vi "FormProductsCluster.vi"() -> ()   [LabVIEW 2013]
panel:
  in  "功能选择":T1
  in  "选项卡控件":T2(tab)
  in  "平均值差":cluster{"limitH":dbl, "unit":string}
  in  "波动值":cluster{"limitH":dbl, "unit":string}
  in  "磨合负载":cluster{"vaule":dbl, "unit":string}
  in  "磨合次数":cluster{"vaule":dbl, "unit":string}
  in  "磨合圈数":cluster{"vaule":dbl, "unit":string}
  in  "检测速度":cluster{"vaule":dbl, "unit":string}
  in  "磨合速度":cluster{"vaule":dbl, "unit":string}
  in  "平均值":T3
  in  "平均值 2":T3
  in  "磨合速度 2":cluster{"vaule":dbl, "unit":string}
  in  "检测速度 2":cluster{"vaule":dbl, "unit":string}
  in  "磨合圈数 2":cluster{"vaule":dbl, "unit":string}
  in  "磨合次数 2":cluster{"vaule":dbl, "unit":string}
  in  "磨合负载 2":cluster{"vaule":dbl, "unit":string}
  in  "波动值 2":cluster{"limitH":dbl, "unit":string}
  in  "平均值差 2":cluster{"limitH":dbl, "unit":string}
  in  "产品选择":bool
  in  "产品删除":bool
  in  "产品更新":bool
  in  "产品注册":bool
  in  "产品":string(combo)
  # "磨合速度"
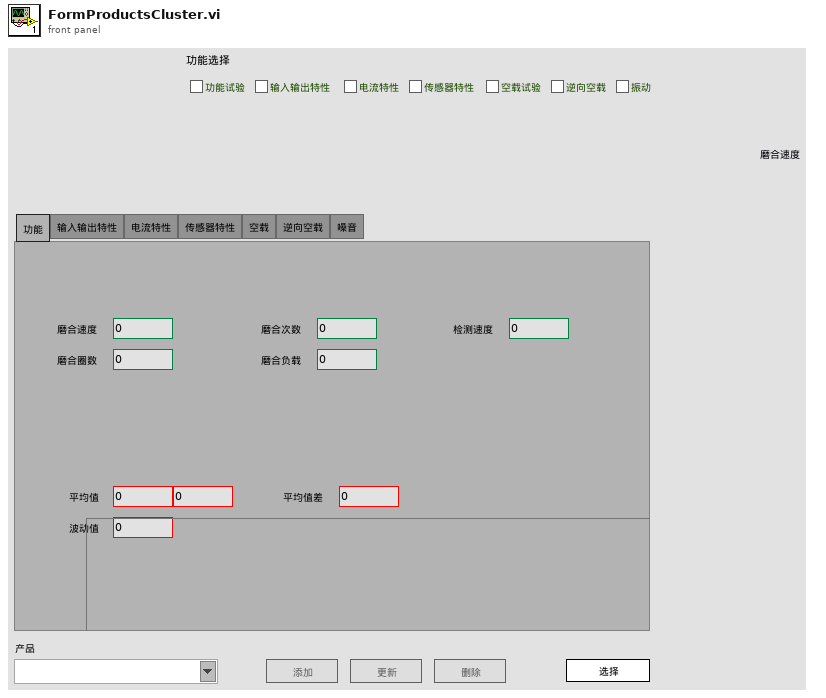
[diagram p1: front panel]
types:
  T1 = cluster{"功能试验":bool, "输入输出特性":bool, "电流特性":bool, "传感器特性":bool, "空载试验":bool, "逆向空载":bool, "振动":bool}
  T2 = enum32{"功能", "输入输出特性", "电流特性", "传感器特性", "空载", "逆向空载", "噪音"}
  T3 = cluster{"limitH":dbl, "limitL":dbl, "unit":string}
  T4 = enum8{"Enabled", "Disabled", "Disabled and Grayed Out"}
  T5 = enum16{"selectdata", "selectsave", "selectlist", "selectshow"}
  T6 = cluster{"userCode":string, "userName":string, "userStatus":string, "connectionMode":string, "takesTime":string, "countDone":string, "countOK":string, "countNG":string, "rigStatus":string, "productsName":string, "partCode1":string, "partCode2":string, "partCode3":string}
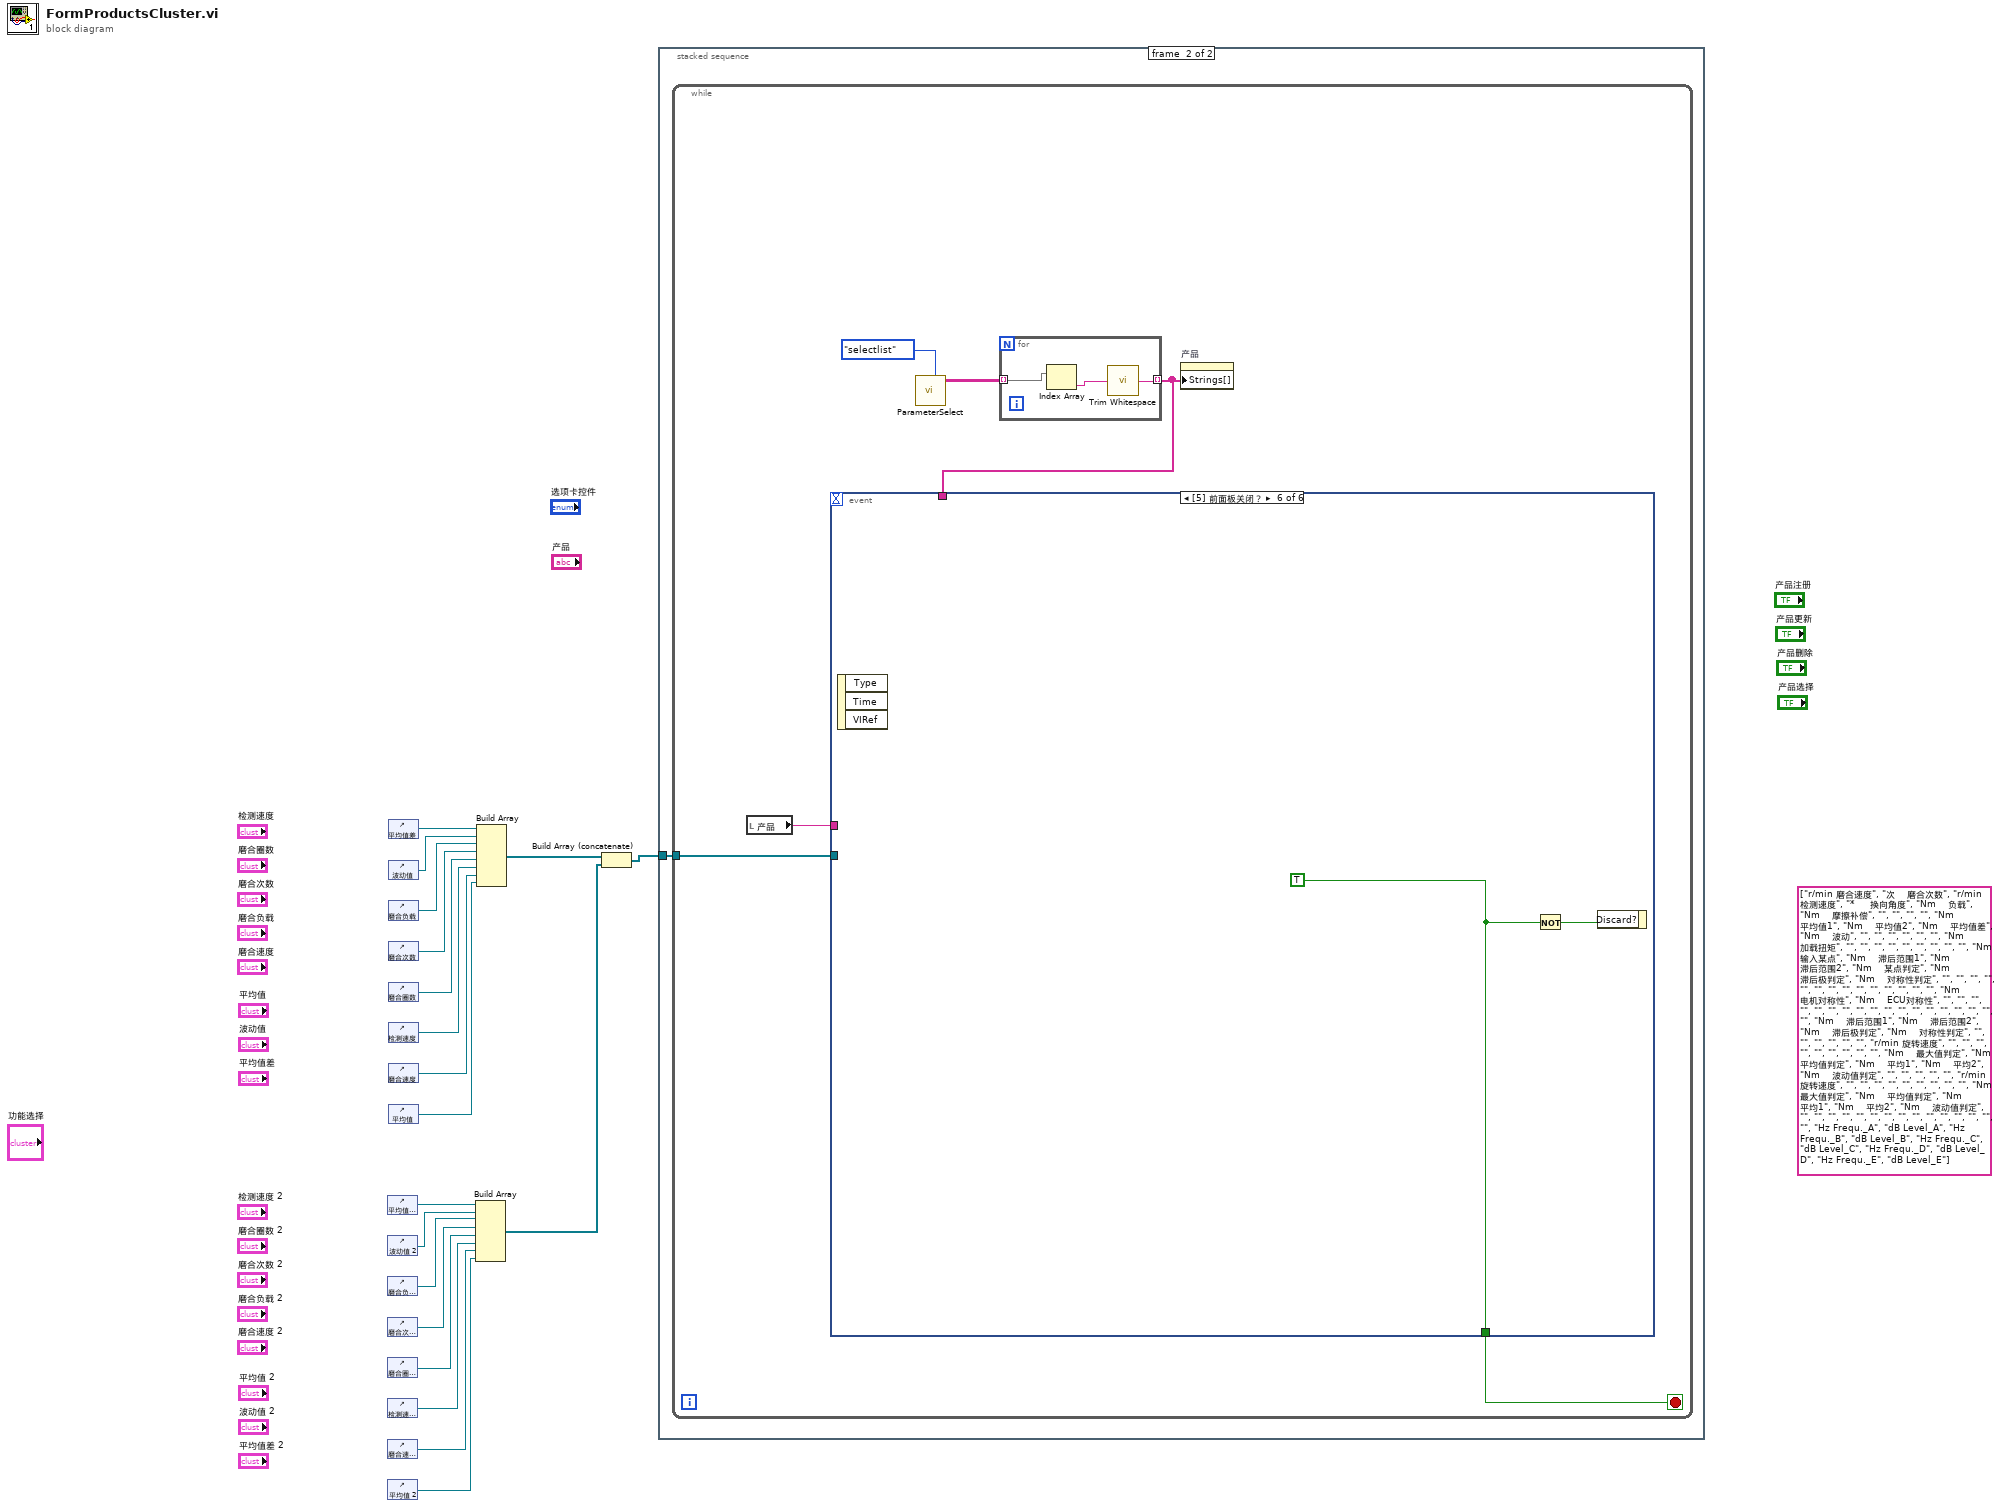
[diagram p0: block diagram]
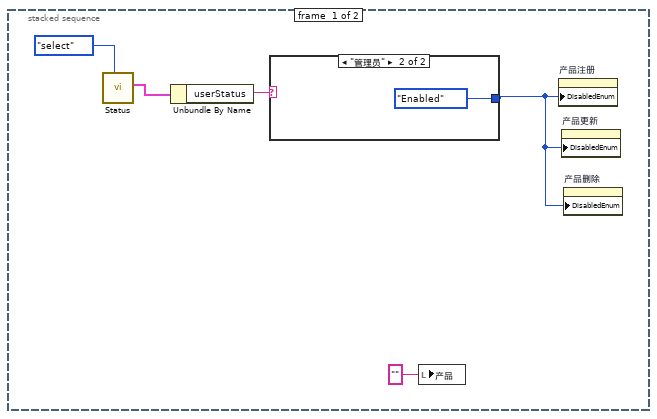
[diagram p2: hidden frame]
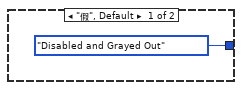
[diagram p3: hidden frame]
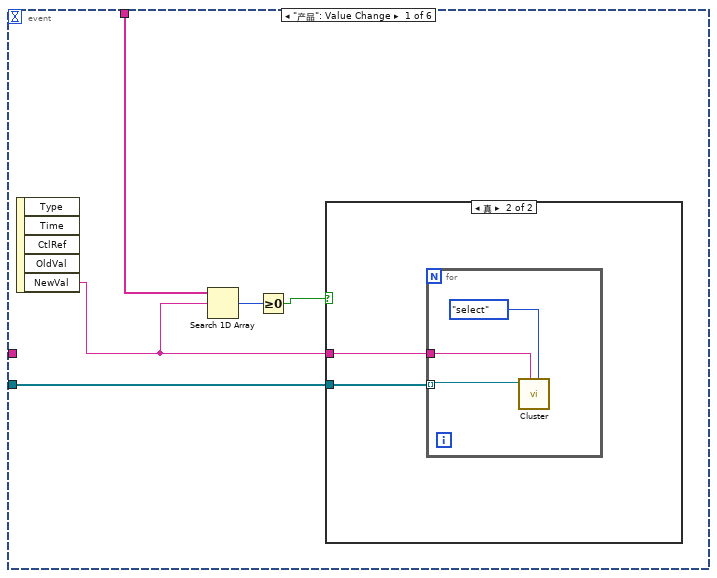
[diagram p4: hidden frame]
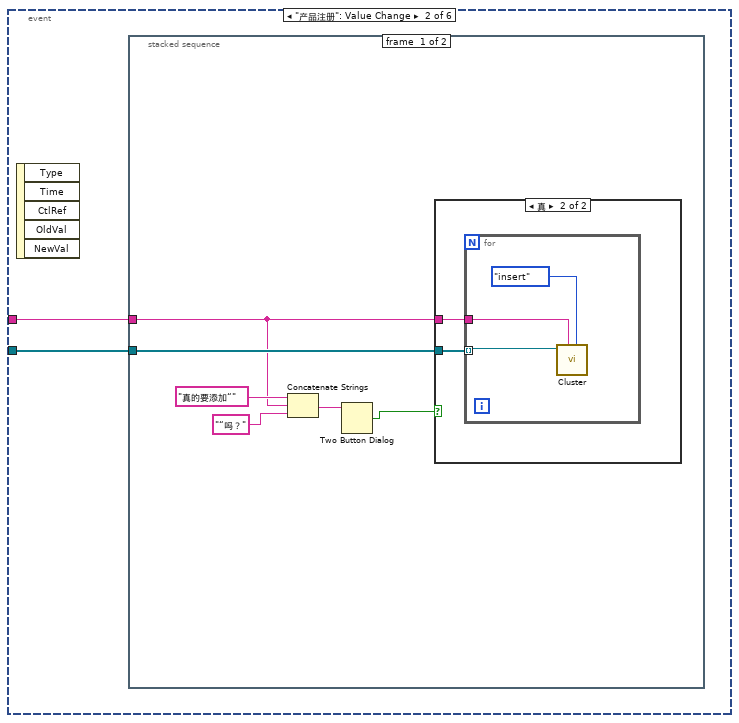
[diagram p6: hidden frame]
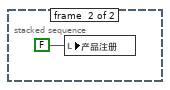
[diagram p8: hidden frame]
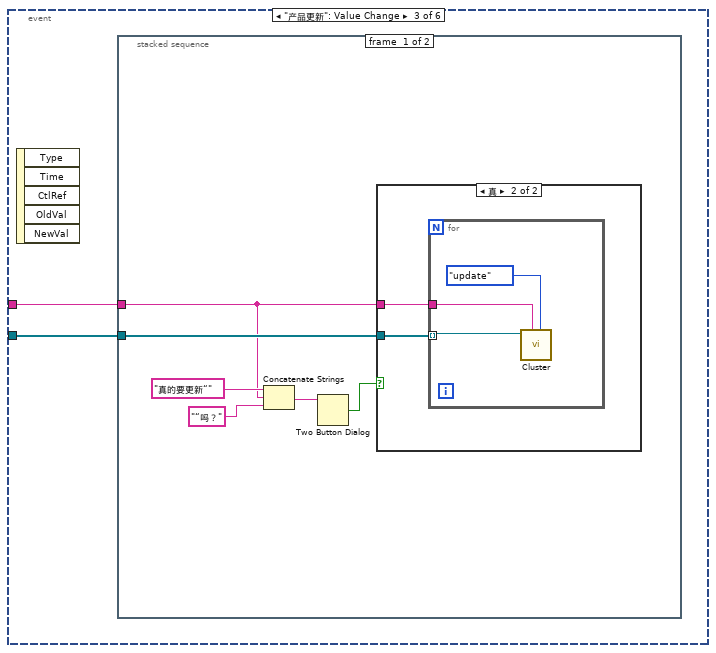
[diagram p9: hidden frame]
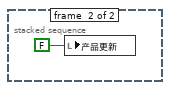
[diagram p11: hidden frame]
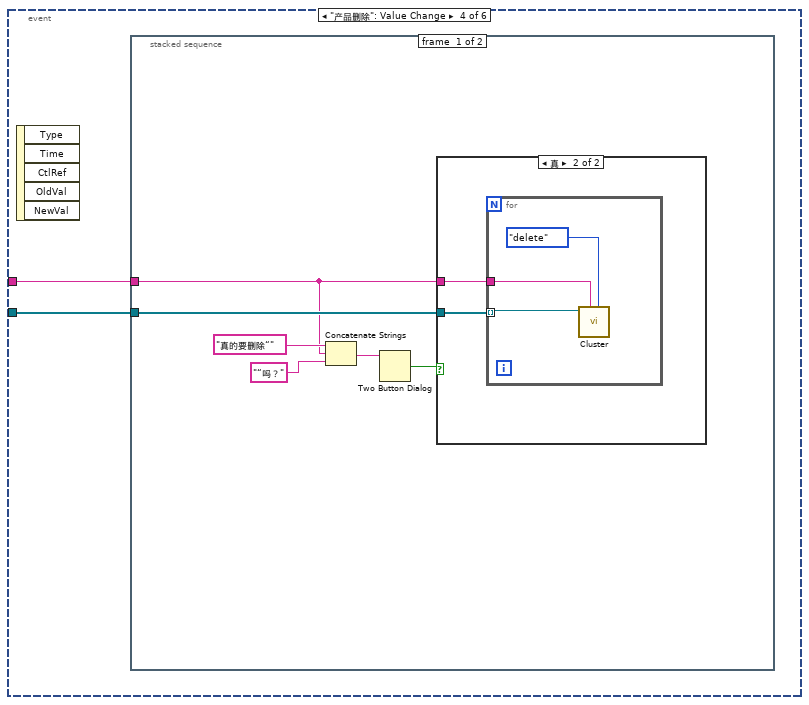
[diagram p12: hidden frame]
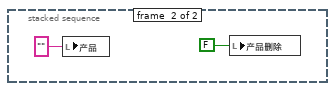
[diagram p14: hidden frame]
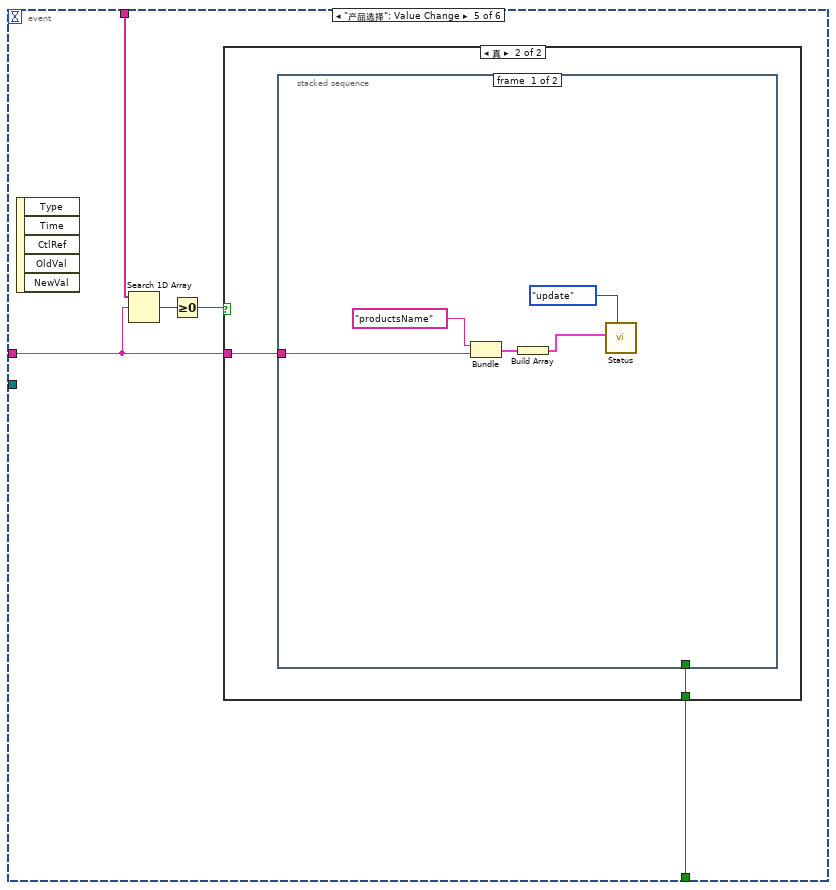
[diagram p15: hidden frame]
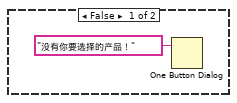
[diagram p16: hidden frame]
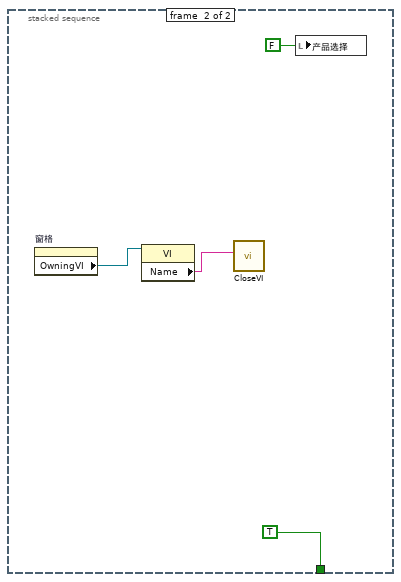
[diagram p17: hidden frame]
diagram:
  (unwired) string[] ["r/min 磨合速度", "次    磨合次数", "r/min 检测速度", "*     换向角度", "Nm    负载", "Nm    摩擦补偿", "", "", "", "", "Nm    平均值1", "Nm    平均值2", "Nm    平均值差", "Nm    波动", "", "", "", "", "", "", "Nm    加载扭矩", "", "", "", "", "", "", "", "", "", "Nm    输入某点", "Nm    滞后范围1", "Nm    滞后范围2", "Nm    某点判定", "Nm    滞后极判定", "Nm    对称性判定", "", "", "", "", "", "", "", "", "", "", "", "", "", "", "Nm    电机对称性", "Nm    ECU对称性", "", "", "", "", "", "", "", "", "", "", "", "", "", "", "", "", "", "", "Nm    滞后范围1", "Nm    滞后范围2", "Nm    滞后极判定", "Nm    对称性判定", "", "", "", "", "", "", "r/min 旋转速度", "", "", "", "", "", "", "", "", "", "Nm    最大值判定", "Nm    平均值判定", "Nm    平均1", "Nm    平均2", "Nm    波动值判定", "", "", "", "", "", "r/min 旋转速度", "", "", "", "", "", "", "", "", "", "Nm    最大值判定", "Nm    平均值判定", "Nm    平均1", "Nm    平均2", "Nm    波动值判定", "", "", "", "", "", "", "", "", "", "", "", "", "", "", "", "Hz Frequ._A", "dB Level_A", "Hz Frequ._B", "dB Level_B", "Hz Frequ._C", "dB Level_C", "Hz Frequ._D", "dB Level_D", "Hz Frequ._E", "dB Level_E"] ("数组")
  n1 = control-ref of="平均值差 2"() -> (w4:refnum<vi>)
  n2 = control-ref of="波动值 2"() -> (w5:refnum<vi>)
  n3 = control-ref of="磨合负载 2"() -> (w6:refnum<vi>)
  n4 = control-ref of="磨合次数 2"() -> (w7:refnum<vi>)
  n5 = control-ref of="磨合圈数 2"() -> (w8:refnum<vi>)
  n6 = control-ref of="检测速度 2"() -> (w9:refnum<vi>)
  n7 = control-ref of="磨合速度 2"() -> (w10:refnum<vi>)
  n8 = control-ref of="平均值 2"() -> (w11:refnum<vi>)
  n9 = control-ref of="平均值差"() -> (w12:refnum<vi>)
  n10 = control-ref of="波动值"() -> (w13:refnum<vi>)
  n11 = control-ref of="磨合负载"() -> (w14:refnum<vi>)
  n12 = control-ref of="磨合次数"() -> (w15:refnum<vi>)
  n13 = control-ref of="磨合圈数"() -> (w16:refnum<vi>)
  n14 = control-ref of="检测速度"() -> (w17:refnum<vi>)
  n15 = control-ref of="磨合速度"() -> (w18:refnum<vi>)
  n16 = control-ref of="平均值"() -> (w19:refnum<vi>)
  n17 = Build Array(w4, w5, w6, w7, w8, w9, w10, w11) -> (w1:refnum<vi>[])
  n18 = Build Array(w12, w13, w14, w15, w16, w17, w18, w19) -> (w2:refnum<vi>[])
  n19 = Build Array (concatenate)(w2, w1) -> (w3:refnum<vi>[])
  n20 = stacked-sequence {
    tunnel: w3 -> [_ w27]
    frame #0 {
      n21 = call "Status.vi"("模式"=enum16{"select", "insert", "update", "delete"}."select") -> ("元素"=w21:T6)  [unwired: 10 in]
      n22 = Unbundle By Name(w21) -> ("userStatus"=w23:string)
      n23 = case shown="\"管理员\"" w23 {
        tunnel: [T4."Disabled and Grayed Out" ("禁用") T4."Enabled" ("禁用")] -> w20
        frame "假", Default {
        }
        frame "管理员" {
        }
      }
      n24 = local write "产品"("" ("y")) -> ()
      n25 = property on="产品注册" class="Bool (严格)"("DisabledEnum"=w20) -> ()  [unwired: 2 in, 2 out]
      n26 = property on="产品更新" class="Bool (严格)"("DisabledEnum"=w20) -> ()  [unwired: 2 in, 2 out]
      n27 = property on="产品删除" class="Bool (严格)"("DisabledEnum"=w20) -> ()  [unwired: 2 in, 2 out]
    }
    frame #1 {
      n28 = while {
        tunnel: w27 -> [w30]
        stop <- w33 stop-if-true
        n29 = local read "产品"() -> (w32:string)
        n30 = call "ParameterSelect.vi"("模式"=T5."selectlist") -> ("dataOutAll"=w29:string[][])  [unwired: 5 in, 5 out]
        n31 = for {
          tunnel: w29 -> [w35] mode=indexing
          tunnel: [w36] -> w31 mode=indexing
          n32 = Index Array(array=w35) -> (element=w34:string)  [unwired: 1 in]
          n33 = call <vilib>:"Trim Whitespace.vi"("string"=w34) -> ("trimmed string"=w36:string)  [unwired: 1 in]
        }
        n34 = event shown="[5] 前面板关闭？" {
          selector: _ -> [_ _ _ _ _ _]
          dyn-events: _ -> [_ _ _ _ _ _]
          timeout: _ -> [_ _ _ _ _ _]
          tunnel: [_ _ _ _ w94 w107] -> w33
          tunnel: w30 -> [w41 w48 w62 w76 _ _]
          tunnel: w32 -> [_ w47 w61 w75 w92 _]
          tunnel: w31 -> [w40 _ _ _ w93 _]
          event "产品": Value Change {
            n35 = event-data() -> ("NewVal"=w38:string)  [unwired: 1 in, 4 out]
            n36 = Search 1D Array(1D array=w40, element=w38) -> (index of element=w39:i32)  [unwired: 1 in]
            n37 = Greater Or Equal To 0?(x=w39) -> (x >= 0?=w37:bool)
            n38 = case shown="真" w37 {
              tunnel: w41 -> [_ w43]
              tunnel: w38 -> [_ w42]
              frame False {
              }
              frame True {
                n39 = for {
                  tunnel: w43 -> [w45] mode=indexing
                  tunnel: w42 -> [w44]
                  n40 = call "Cluster.vi"("模式 2"=enum16{"select", "insert", "update", "delete"}."select", "productsName"=w44, "limit"=w45) -> ()  [unwired: 9 in]
                }
              }
            }
          }
          event "产品注册": Value Change {
            n41 = event-data() -> ()  [unwired: 1 in, 5 out]
            n42 = stacked-sequence {
              tunnel: w48 -> [w54 _]
              tunnel: w47 -> [w49 _]
              frame #0 {
                n43 = Concatenate Strings("真的要添加“" ("消息"), w49, "“吗？" ("消息")) -> (w51:string)
                n44 = Two Button Dialog(message=w51) -> (T button?=w50:bool)  [unwired: 2 in]
                n45 = case shown="真" w50 {
                  tunnel: w54 -> [_ w56]
                  tunnel: w49 -> [_ w55]
                  frame False {
                  }
                  frame True {
                    n46 = for {
                      tunnel: w56 -> [w57] mode=indexing
                      tunnel: w55 -> [w58]
                      n47 = call "Cluster.vi"("模式 2"=enum16{"select", "insert", "update", "delete"}."insert", "productsName"=w58, "limit"=w57) -> ()  [unwired: 9 in]
                    }
                  }
                }
              }
              frame #1 {
                n48 = local write "产品注册"(FALSE ("产品注册")) -> ()
              }
            }
          }
          event "产品更新": Value Change {
            n49 = event-data() -> ()  [unwired: 1 in, 5 out]
            n50 = stacked-sequence {
              tunnel: w62 -> [w68 _]
              tunnel: w61 -> [w63 _]
              frame #0 {
                n51 = Concatenate Strings("真的要更新“" ("消息"), w63, "“吗？" ("消息")) -> (w65:string)
                n52 = Two Button Dialog(message=w65) -> (T button?=w64:bool)  [unwired: 2 in]
                n53 = case shown="真" w64 {
                  tunnel: w68 -> [_ w70]
                  tunnel: w63 -> [_ w69]
                  frame False {
                  }
                  frame True {
                    n54 = for {
                      tunnel: w70 -> [w71] mode=indexing
                      tunnel: w69 -> [w72]
                      n55 = call "Cluster.vi"("模式 2"=enum16{"select", "insert", "update", "delete"}."update", "productsName"=w72, "limit"=w71) -> ()  [unwired: 9 in]
                    }
                  }
                }
              }
              frame #1 {
                n56 = local write "产品更新"(FALSE ("产品注册")) -> ()
              }
            }
          }
          event "产品删除": Value Change {
            n57 = event-data() -> ()  [unwired: 1 in, 5 out]
            n58 = stacked-sequence {
              tunnel: w76 -> [w82 _]
              tunnel: w75 -> [w77 _]
              frame #0 {
                n59 = Concatenate Strings("真的要删除“" ("消息"), w77, "“吗？" ("消息")) -> (w79:string)
                n60 = Two Button Dialog(message=w79) -> (T button?=w78:bool)  [unwired: 2 in]
                n61 = case shown="真" w78 {
                  tunnel: w82 -> [_ w84]
                  tunnel: w77 -> [_ w83]
                  frame False {
                  }
                  frame True {
                    n62 = for {
                      tunnel: w84 -> [w87] mode=indexing
                      tunnel: w83 -> [w85]
                      n63 = call "Cluster.vi"("模式 2"=enum16{"select", "insert", "update", "delete"}."delete", "productsName"=w85, "limit"=w87) -> ()  [unwired: 9 in]
                    }
                  }
                }
              }
              frame #1 {
                n64 = local write "产品"("" ("products_name_in")) -> ()
                n65 = local write "产品删除"(FALSE ("产品删除")) -> ()
              }
            }
          }
          event "产品选择": Value Change {
            n66 = event-data() -> ()  [unwired: 1 in, 5 out]
            n67 = Search 1D Array(1D array=w93, element=w92) -> (index of element=w91:i32)  [unwired: 1 in]
            n68 = Greater Or Equal To 0?(x=w91) -> (x >= 0?=w90:bool)
            n69 = case shown="真" w90 {
              tunnel: [_ w97] -> w94
              tunnel: w92 -> [_ w96]
              frame False {
                n70 = One Button Dialog(message="没有你要选择的产品！" ("消息")) -> ()  [unwired: 1 in, 1 out]
              }
              frame True {
                n71 = stacked-sequence {
                  tunnel: w96 -> [w100 _]
                  tunnel: [_ TRUE ("产品删除")] -> w97
                  frame #0 {
                    n72 = Bundle("name"="productsName", "产品"=w100) -> (w99:cluster{"name":string, "产品":string})  [unwired: 1 in]
                    n73 = Build Array(w99) -> (w98:cluster{"name":string, "产品":string}[])
                    n74 = call "Status.vi"("模式"=enum16{"select", "insert", "update", "delete"}."update", "nameData"=w98) -> ()  [unwired: 9 in, 1 out]
                  }
                  frame #1 {
                    n75 = property on="窗格" class="Pane"() -> ("OwningVI"=w104:refnum<vi>)  [unwired: 2 in, 2 out]
                    n76 = property on="属性节点" class="VI"(reference=w104) -> ("Name"=w103:string)  [unwired: 1 in, 2 out]
                    n77 = call "CloseVI.vi"("名称或相对路径"=w103) -> ()  [unwired: 10 in, 1 out]
                    n78 = local write "产品选择"(FALSE ("产品删除")) -> ()
                  }
                }
              }
            }
          }
          event Panel Close? {
            w107 = TRUE
            n79 = event-data() -> ()  [unwired: 1 in, 3 out]
            n80 = Not(x=w107) -> (.not. x?=w108:bool)
            n81 = event-data("Discard?"=w108) -> ()  [unwired: 1 in, 1 out]
          }
        }
        n82 = property on="产品" class="CmbBox"("Strings[]"=w31) -> ()  [unwired: 2 in, 2 out]
      }
    }
  }
